vi "Query Number Of Stored Points.vi"(8 "Error In (no error)":errorcluster, 11 "VISA Resource Name":refnum<visa-resource-name>) -> (0 "Error Out":errorcluster, 2 "Number Of Points":i16, 3 "VISA Resource Name Out":refnum<visa-resource-name>)   [LabVIEW 2010, in "Stanford Research 844.lvlib"]
doc: "This VI queries the number of points currently stored in the buffer. \n\nNote: The same number of points is stored from each display. If the buffer is reset, then 0 is returned."
uses:
  <instrlib>/Stanford Research 844/Stanford Research 844.lvlib
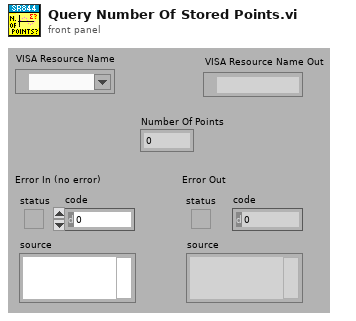
[diagram p1: front panel]
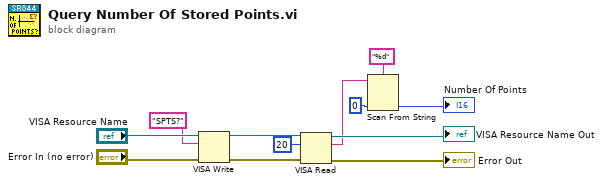
[diagram p0: block diagram]
diagram:
  n1 = VISA Write(VISA resource name="VISA Resource Name", write buffer="SPTS?" ("write buffer (\"\")"), error in (no error)="Error In (no error)") -> (VISA resource name out=w9:refnum<visa-resource-name>, error out=w10:errorcluster)  [unwired: 1 out]
  n2 = VISA Read(VISA resource name=w9, byte count=u32 20 ("byte count (0)"), error in (no error)=w10) -> (VISA resource name out=→"VISA Resource Name Out":refnum<visa-resource-name>, read buffer=w3:string, error out=→"Error Out":errorcluster)  [unwired: 1 out]
  n3 = Scan From String(format string="%d", input string=w3, default 1=0 ("default value 1")) -> (output 1=→"Number Of Points":i32)  [unwired: 2 in, 3 out]
